vi "Collect 106F Data.vi"(1 "Boolean":bool, 2 "Lights ON":bool, 3 "Boolean 2":bool, 4 "Accept Power Failure Delay":bool, 5 "Accept Watchdog Delay":bool, 6 "Boolean 3":bool) -> (0 "String":string)   [LabVIEW 2009]
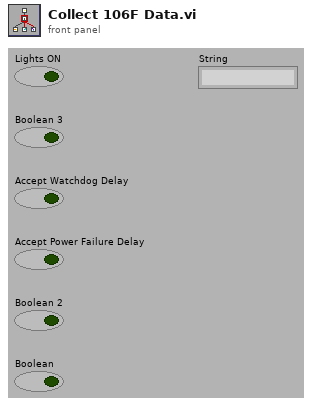
[diagram p1: front panel]
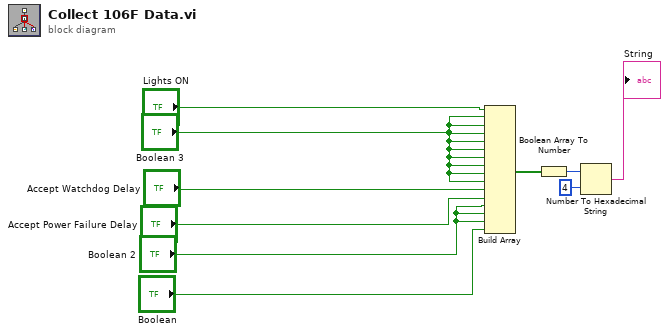
[diagram p0: block diagram]
diagram:
  n1 = Build Array("Lights ON", "Boolean 3", "Boolean 3", "Boolean 3", "Boolean 3", "Boolean 3", "Boolean 3", "Boolean 3", "Boolean 3", "Boolean 3", "Accept Watchdog Delay", "Accept Power Failure Delay", "Boolean 2", "Boolean 2", "Boolean 2", "Boolean") -> (w4:bool[])
  n2 = Boolean Array To Number(Boolean array=w4) -> (number=w1:u32)
  n3 = Number To Hexadecimal String(1:i16 4 ("width (-)"), 2:w1) -> (0:→"String":string)
